vi "Config.Gui.Stop.vi"(8 "error in":errorcluster, 11 "Ref":refnum<vi>) -> (0 "error out":errorcluster)   [LabVIEW 2013]
uses:
  Config.Gui.Action.ctl
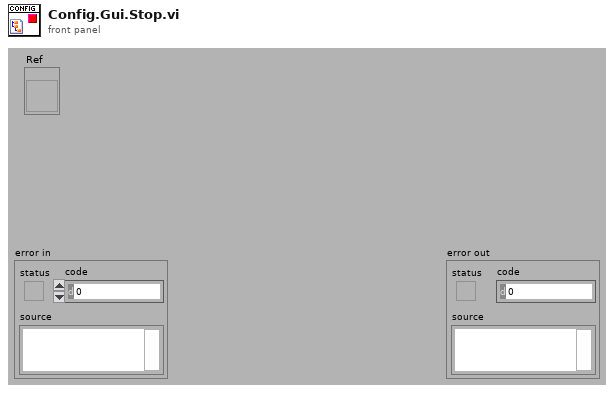
[diagram p1: front panel]
types:
  T1 = typedef "Config.Gui.Action.ctl" = enum32{"idle", "constructor", "destructor", "--- Config.Gui ---", "read from global", "write to global", "write"}
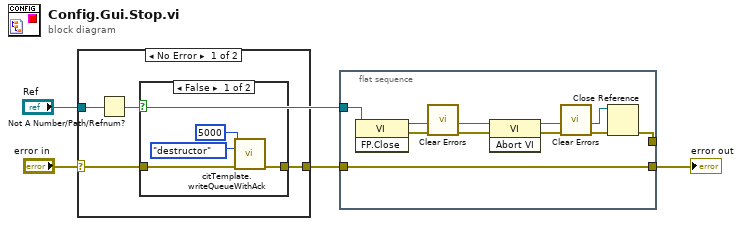
[diagram p0: block diagram]
diagram:
  n1 = case shown="No Error" "error in" {
    selector: "error in" -> [w8 w14]
    tunnel: [w5 w14] -> w3
    tunnel: "Ref" -> [w6 _]
    frame No Error {
      n2 = Not A Number/Path/Refnum?(number/path/refnum=w6) -> (NaN/Path/Refnum?=w7:bool)
      n3 = case shown="False" w7 {
        tunnel: w8 -> [w11 w13]
        tunnel: [w10 w13] -> w5
        frame False {
          n4 = call "citTemplate.writeQueueWithAck.vi"("timeout ms (-1)"=5000, "event in"=Config.Gui.Action."destructor" ("Action"), "error in (no error)"=w11) -> ("error out"=w10:errorcluster)  [unwired: 10 in, 2 out]
        }
        frame True {
        }
      }
    }
    frame Error {
    }
  }
  n5 = flat-sequence {
    tunnel: w3 -> [w23]
    tunnel: "Ref" -> [w16]
    tunnel: [w23] -> w2
    tunnel: [w22] -> _
    frame #0 {
      n6 = invoke class="VI" method="FP.Close"(reference=w16) -> (reference out=w20:refnum<vi>, error out=w21:errorcluster)  [unwired: 2 in, 1 out]
      n7 = call <vilib>:"Clear Errors.vi"("error in (no error)"=w21) -> ("error out"=w19:errorcluster)  [unwired: 6 in]
      n8 = invoke class="VI" method="Abort VI"(reference=w20, error in=w19) -> (reference out=w15:refnum<vi>, error out=w18:errorcluster)  [unwired: 1 in, 1 out]
      n9 = call <vilib>:"Clear Errors.vi"("error in (no error)"=w18) -> ("error out"=w17:errorcluster)  [unwired: 6 in]
      n10 = Close Reference(reference=w15, error in (no error)=w17) -> (error out=w22:errorcluster)
    }
  }
  "error out" <- w2
